vi "Get Intake Queue.vi"(8 "error in":errorcluster) -> (0 "error out":errorcluster, 3 "queue out":refnum<queue>)   [LabVIEW 2016, in "Intake.lvlib"]
uses:
  Intake.lvlib
  Typedef/Intake Msg.ctl
  Typedef/Intake Command.ctl
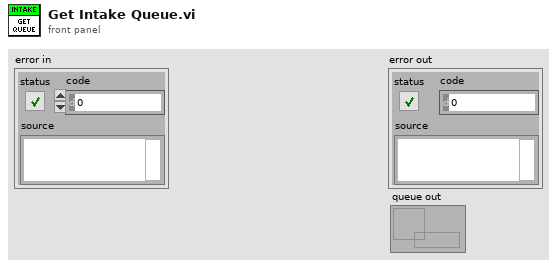
[diagram p1: front panel]
types:
  T1 = typedef "Intake.lvlib/Intake Msg.ctl" = cluster{"Cmd":T2, "Variant":variant}
  T2 = typedef "Intake.lvlib/Intake Command.ctl" = enum16{"Gear On", "Gear Off", "Gear Reverse", "Gear Release", "Fuel Deploy", "Fuel Retract", "Fuel Agitate", "Fuel Reverse"}
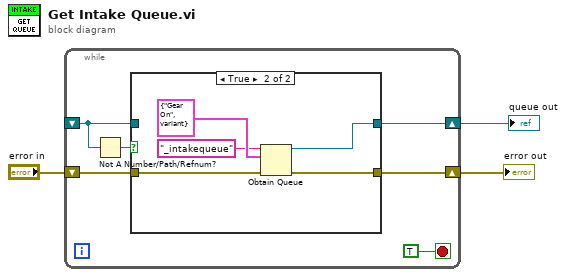
[diagram p0: block diagram]
diagram:
  n1 = while {
    shift-right: [w8] -> w2
    shift-left: "error in" -> [w9]
    shift-right: [w7] -> w1
    shift-left: _ -> [w4]
    stop <- TRUE stop-if-true
    n2 = Not A Number/Path/Refnum?(number/path/refnum=w4) -> (NaN/Path/Refnum?=w5:bool)
    n3 = case shown="True" w5 {
      tunnel: w9 -> [w10 w14]
      tunnel: [w10 w13] -> w8
      tunnel: [w11 w12] -> w7
      tunnel: w4 -> [w11 _]
      frame False {
      }
      frame True {
        n4 = Obtain Queue(name (unnamed)="_intakequeue", element data type=T1 {"Cmd"=enum."Gear On", "Variant"=variant}, error in (no error)=w14) -> (queue out=w12:refnum<queue>, error out=w13:errorcluster)  [unwired: 2 in, 1 out]
      }
    }
  }
  "error out" <- w2
  "queue out" <- w1
